vi "UTIL Detect Stim.vi"(7 "Predicted State":i32, 8 "Min Duration":dbl, 9 "Target State":u16, 10 "Previous Stim State":bool, 11 "Detection Duration In":dbl) -> (0 "Detection":bool, 2 "Stim State Out":bool, 3 "Detection Duration Out":dbl)   [LabVIEW 2017]
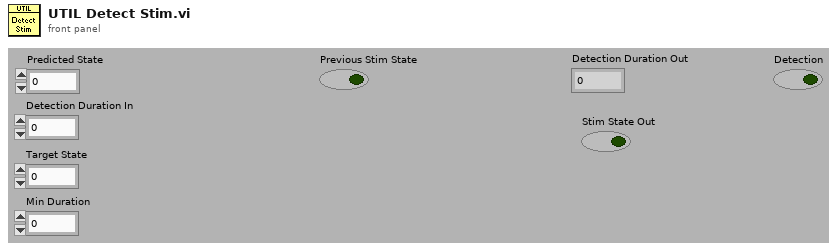
[diagram p1: front panel]
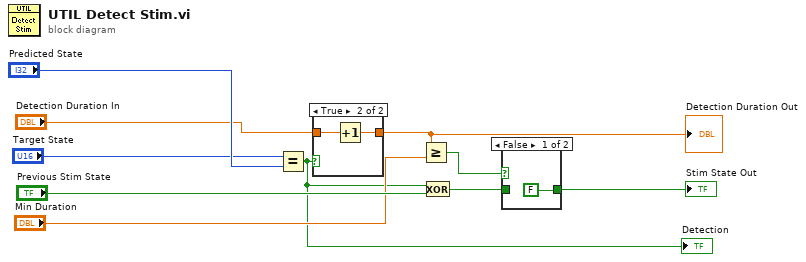
[diagram p0: block diagram]
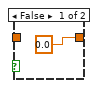
[diagram p3: hidden frame]
diagram:
  n1 = Equal?(x="Target State", y="Predicted State") -> (x = y?=w1:bool)
  "Detection" <- w1
  n2 = case shown="True" w1 {
    tunnel: "Detection Duration In" -> [_ w13]
    tunnel: [0.0 ("element") w12] -> w4
    frame False {
    }
    frame True {
      n3 = Increment(x=w13) -> (x+1=w12:dbl)
    }
  }
  "Detection Duration Out" <- w4
  n4 = Greater Or Equal?(x=w4, y="Min Duration") -> (x >= y?=w2:bool)
  n5 = Exclusive Or(1:"Previous Stim State", 2:w1) -> (0:w9:bool)
  n6 = case shown="False" w2 {
    tunnel: [FALSE w15] -> w10
    tunnel: w9 -> [_ w15]
    frame False {
    }
    frame True {
    }
  }
  "Stim State Out" <- w10
